vi "six legs 1.vi"   [LabVIEW 2010, in "Six Legs.lvrbt"]
uses:
  Six Legs.lvrbt
  <vilib>/NXT/Block Support/NXT_InputPort.ctl
  <vilib>/NXT/Subs/MotorOutput.ctl
  <vilib>/NXT/Dual Mode Library/Sensors/Sonar_cm.vi
  <vilib>/NXT/Dual Mode Library/Sensors/Touch_Pressed.vi
  <vilib>/NXT/Dual Mode Library/Motors/Rotation.vi
  <vilib>/NXT/Dual Mode Library/Motors/ResetMotor.vi
types:
  T1 = typedef "NXT_InputPort.ctl" = u8
  T2 = typedef "LVHSConnector.ctl" = cluster{"Hardware":string, "Flattened String":string}
  T3 = typedef "MotorOutput.ctl" = u8
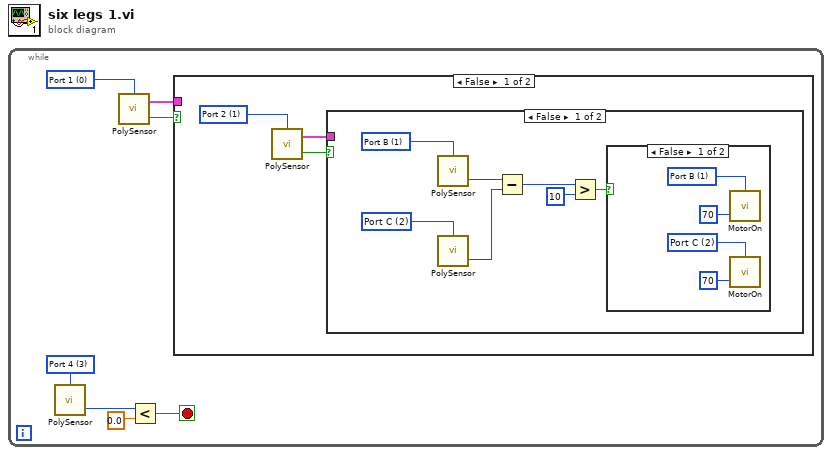
[diagram p0: block diagram]
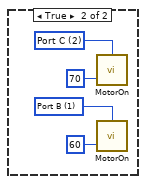
[diagram p2: hidden frame]
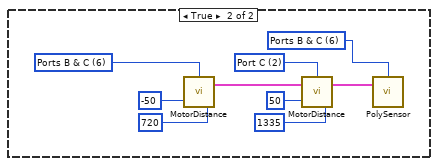
[diagram p3: hidden frame]
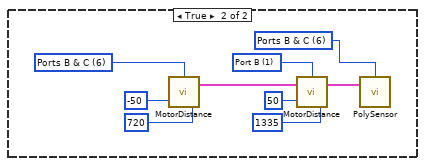
[diagram p4: hidden frame]
diagram:
  n1 = while {
    stop <- w2 stop-if-true
    w1 = T1 3 items=["Port 1", "Port 2", "Port 3", "Port 4"] ("Port (Port 4)")
    w7 = T1 0 items=["Port 1", "Port 2", "Port 3", "Port 4"] ("Port (Port 1)")
    n2 = call-poly <vilib>:"PolySensor.vi"("Port (Port 4)"=w1) -> ("Distance (cm)"=w3:i16)  [unwired: 2 in, 1 out]
    n3 = call-poly <vilib>:"PolySensor.vi"("Port (Port 1)"=w7) -> ("Yes / No"=w5:bool, "NXT"=w6:T2)  [unwired: 2 in]
    n4 = Less?(x=w3, y=0.0) -> (x < y?=w2:bool)
    n5 = case shown="False" w5 {
      tunnel: w6 -> [_ _]
      frame False {
        w10 = T1 1 items=["Port 1", "Port 2", "Port 3", "Port 4"] ("Port (Port 1)")
        n6 = call-poly <vilib>:"PolySensor.vi"("Port (Port 1)"=w10) -> ("Yes / No"=w8:bool, "NXT"=w9:T2)  [unwired: 2 in]
        n7 = case shown="False" w8 {
          tunnel: w9 -> [_ _]
          frame False {
            w16 = T3 2 items=["Port A"=0, "Port B"=1, "Port C"=2, "Ports A & B"=4, "Ports A & C"=5, "Ports B & C"=6, "All Ports"=3] ("Port (All Ports)")
            w17 = T3 1 items=["Port A"=0, "Port B"=1, "Port C"=2, "Ports A & B"=4, "Ports A & C"=5, "Ports B & C"=6, "All Ports"=3] ("Port (All Ports)")
            n8 = call-poly <vilib>:"PolySensor.vi"("Port (Port A)"=w17) -> ("Angle of Rotation"=w15:i32)  [unwired: 2 in, 1 out]
            n9 = call-poly <vilib>:"PolySensor.vi"("Port (Port A)"=w16) -> ("Angle of Rotation"=w14:i32)  [unwired: 2 in, 1 out]
            n10 = Subtract(x=w15, y=w14) -> (x-y=w13:i32)
            n11 = Greater?(x=w13, y=10) -> (0:w11:bool)
            n12 = case shown="False" w11 {
              frame False {
                w19 = T3 2 items=["Port A"=0, "Port B"=1, "Port C"=2, "Ports A & B"=4, "Ports A & C"=5, "Ports B & C"=6, "All Ports"=3] ("Output Port (All Ports)")
                w21 = T3 1 items=["Port A"=0, "Port B"=1, "Port C"=2, "Ports A & B"=4, "Ports A & C"=5, "Ports B & C"=6, "All Ports"=3] ("Output Port (All Ports)")
                n13 = call <vilib>:"MotorOn.vi"("Power (75)"=70, "Output Port (All Ports)"=w21) -> ()  [unwired: 2 in, 1 out]
                n14 = call <vilib>:"MotorOn.vi"("Power (75)"=70, "Output Port (All Ports)"=w19) -> ()  [unwired: 2 in, 1 out]
              }
              frame True {
                w24 = T3 2 items=["Port A"=0, "Port B"=1, "Port C"=2, "Ports A & B"=4, "Ports A & C"=5, "Ports B & C"=6, "All Ports"=3] ("Output Port (All Ports)")
                w25 = T3 1 items=["Port A"=0, "Port B"=1, "Port C"=2, "Ports A & B"=4, "Ports A & C"=5, "Ports B & C"=6, "All Ports"=3] ("Output Port (All Ports)")
                n15 = call <vilib>:"MotorOn.vi"("Power (75)"=70, "Output Port (All Ports)"=w24) -> ()  [unwired: 2 in, 1 out]
                n16 = call <vilib>:"MotorOn.vi"("Power (75)"=60, "Output Port (All Ports)"=w25) -> ()  [unwired: 2 in, 1 out]
              }
            }
          }
          frame True {
            w29 = T3 2 items=["Port A"=0, "Port B"=1, "Port C"=2, "Ports A & B"=4, "Ports A & C"=5, "Ports B & C"=6, "All Ports"=3] ("Output Port (All Ports)")
            w33 = T3 6 items=["Port A"=0, "Port B"=1, "Port C"=2, "Ports A & B"=4, "Ports A & C"=5, "Ports B & C"=6, "All Ports"=3] ("Output Port (All Ports)")
            w26 = T3 6 items=["Port A"=0, "Port B"=1, "Port C"=2, "Ports A & B"=4, "Ports A & C"=5, "Ports B & C"=6, "All Ports"=3] ("Port (All Ports)")
            n17 = call <vilib>:"MotorDistance.vi"("Power (75)"=-50, "Angle of Rotation (360)"=720, "Output Port (All Ports)"=w33) -> ("NXT"=w28:T2)  [unwired: 1 in]
            n18 = call <vilib>:"MotorDistance.vi"("Power (75)"=50, "Angle of Rotation (360)"=1335, "NXT"=w28, "Output Port (All Ports)"=w29) -> ("NXT"=w27:T2)
            n19 = call-poly <vilib>:"PolySensor.vi"("NXT"=w27, "Port (All Ports)"=w26) -> ()  [unwired: 2 in, 1 out]
          }
        }
      }
      frame True {
        w37 = T3 1 items=["Port A"=0, "Port B"=1, "Port C"=2, "Ports A & B"=4, "Ports A & C"=5, "Ports B & C"=6, "All Ports"=3] ("Output Port (All Ports)")
        w41 = T3 6 items=["Port A"=0, "Port B"=1, "Port C"=2, "Ports A & B"=4, "Ports A & C"=5, "Ports B & C"=6, "All Ports"=3] ("Output Port (All Ports)")
        w43 = T3 6 items=["Port A"=0, "Port B"=1, "Port C"=2, "Ports A & B"=4, "Ports A & C"=5, "Ports B & C"=6, "All Ports"=3] ("Port (All Ports)")
        n20 = call <vilib>:"MotorDistance.vi"("Power (75)"=-50, "Angle of Rotation (360)"=720, "Output Port (All Ports)"=w41) -> ("NXT"=w36:T2)  [unwired: 1 in]
        n21 = call <vilib>:"MotorDistance.vi"("Power (75)"=50, "Angle of Rotation (360)"=1335, "NXT"=w36, "Output Port (All Ports)"=w37) -> ("NXT"=w35:T2)
        n22 = call-poly <vilib>:"PolySensor.vi"("NXT"=w35, "Port (All Ports)"=w43) -> ()  [unwired: 2 in, 1 out]
      }
    }
  }
